vi "Validate Client Names.vi"(8 "error in (no error)":errorcluster, 10 "project ref":refnum<vi>, 11 "multicolumnListbox in":refnum<vi>) -> (0 "error out":errorcluster, 2 "warning?":bool, 3 "multicolumnListbox out":refnum<vi>)   [LabVIEW 2021, in "MeasurementClient Editor.lvlib"]
uses:
  MeasurementClient Editor.lvlib
  <vilib>/Utility/miscctls.llb/LVRowAndColumnTypeDef.ctl
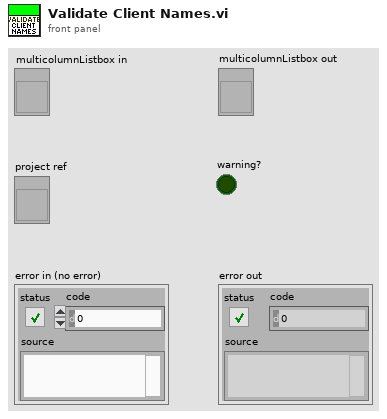
[diagram p1: front panel]
types:
  T1 = typedef "LVRowAndColumnTypeDef.ctl" = cluster{"Row":i32, "Column":i32}
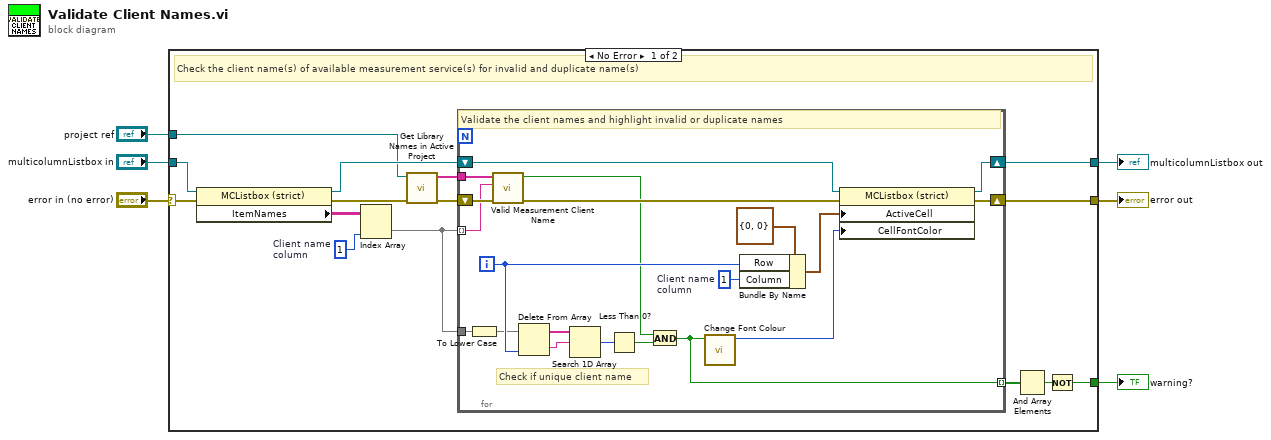
[diagram p0: block diagram]
diagram:
  n1 = case shown="No Error" "error in (no error)" {
    selector: "error in (no error)" -> [w20 w43]
    tunnel: "multicolumnListbox in" -> [w21 w42]
    tunnel: [w17 w43] -> w4
    tunnel: [w16 w42] -> w3
    tunnel: [w14 _] -> w2
    tunnel: "project ref" -> [w12 _]
    frame No Error {
      w19 = 1  # Client name column
      # "Check the client name(s) of available measurement service(s) for invalid and duplicate name(s)"
      n2 = property class="MCListbox (strict)"(reference=w21, error in=w20) -> (reference out=w18:refnum<vi>, error out=w8:errorcluster, "ItemNames"=w9:string[][])
      n3 = Index Array(array=w9, index (col)=w19) -> (element=w10:string[])  [unwired: 1 in]
      n4 = call "Get Library Names in Active Project.vi"("error in (no error)"=w8, "project ref"=w12) -> ("error out"=w13:errorcluster, "library names"=w11:string[])  [unwired: 8 in]
      n5 = for {
        shift-right: [w34] -> w17
        shift-left: w13 -> [w41]
        shift-right: [w33] -> w16
        shift-left: w18 -> [w39]
        tunnel: [w22] -> w7 mode=indexing
        tunnel: w11 -> [w25]
        tunnel: w10 -> [w24] mode=indexing
        tunnel: w10 -> [w23]
        i -> [w30]
        w36 = 1  # Client name column
        # "Check if unique client name"
        # "Validate the client names and highlight invalid or duplicate names"
        n6 = To Lower Case(string=w23) -> (all lower case string=w26:string[])
        n7 = call "Valid Measurement Client Name.vi"("error in"=w41, "requested client name"=w24, "library names"=w25) -> ("error out"=w40:errorcluster, "valid name?"=w27:bool)  [unwired: 7 in]
        n8 = Delete From Array(array=w26, index=w30) -> (deleted portion=w31:string, array with subset deleted=w32:string[])  [unwired: 1 in]
        n9 = Search 1D Array(1D array=w32, element=w31) -> (index of element=w29:i32)  [unwired: 1 in]
        n10 = Less Than 0?(x=w29) -> (x < 0?=w28:bool)
        n11 = And(x=w27, y=w28) -> (x .and. y?=w22:bool)
        n12 = call "Change Font Colour.vi"("valid?"=w22) -> ("font colour"=w35:u32)  [unwired: 10 in]
        n13 = Bundle By Name(cluster=T1 {"Row"=0, "Column"=0} ("Active Cell:Active Cell"), "Row"=w30, "Column"=w36) -> (w37:T1)
        n14 = property class="MCListbox (strict)"(reference=w39, error in=w40, "ActiveCell"=w37, "CellFontColor"=w35) -> (reference out=w33:refnum<vi>, error out=w34:errorcluster)
      }
      n15 = And Array Elements(Boolean array=w7) -> (logical AND=w15:bool)
      n16 = Not(x=w15) -> (.not. x?=w14:bool)
    }
    frame Error {
      # "Pass"
    }
  }
  "error out" <- w4
  "multicolumnListbox out" <- w3
  "warning?" <- w2
